vi "Check Elf in Direction.vi"(7 "List No Center Out":T1[](array[typedef]), 10 "Direction":T1, 11 "Elf Present Array":T2[](array[typedef])) -> (2 "Direction Loc Out":T1, 3 "Elf Found Out":bool)   [LabVIEW 2020]
uses:
  ENUM_Location Direction.ctl
  RB ENUM_Spot ID.ctl
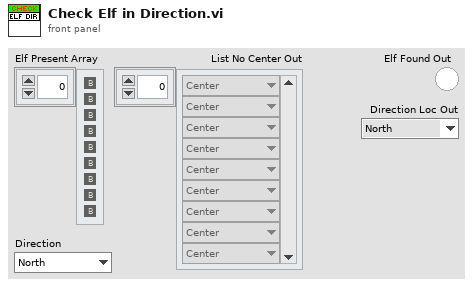
[diagram p1: front panel]
types:
  T1 = typedef "ENUM_Location Direction.ctl" = enum16{"North", "North-East", "East", "South-East", "South", "South-West", "West", "North-West", "Center"}
  T2 = typedef "RB ENUM_Spot ID.ctl" = enum32{"Blank", "ELF", "Proposed"}
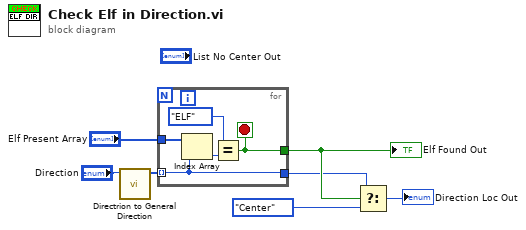
[diagram p0: block diagram]
diagram:
  n1 = call "Directrion to General Direction.vi"("Direction"="Direction") -> ("General Direction"=w6:T1[])  [unwired: 10 in]
  n2 = for {
    tunnel: w6 -> [w8] mode=indexing
    tunnel: "Elf Present Array" -> [w12]
    tunnel: [w9] -> w4
    tunnel: [w8] -> w3
    stop <- w9 stop-if-true
    n3 = Index Array(array=w12, index=w8) -> (element=w11:T2)
    n4 = Equal?(x=RB_ENUM_Spot_ID."ELF" ("y"), y=w11) -> (x = y?=w9:bool)
  }
  "Elf Found Out" <- w4
  n5 = Select(t=w3, s=w4, f=ENUM_Location_Direction."Center") -> (s? t:f=→"Direction Loc Out":T1)
